vi "Get State.vi"(8 "error in (no error)":errorcluster, 11 "Tektronix Driver in":refnum<class "Tektronix Driver.lvclass">) -> (0 "error out":errorcluster, 1 "Data ready":bool, 2 "Armed":bool, 3 "Tektronix Driver out":refnum<class "Tektronix Driver.lvclass">, 4 "Availiable Samples":u32, 5 "Finished":bool)   [LabVIEW 2020, in "Tektronix Driver.lvclass"]
uses:
  Tektronix Driver.lvclass
  Tektronix Driver.lvclass/Tektronix Driver.ctl
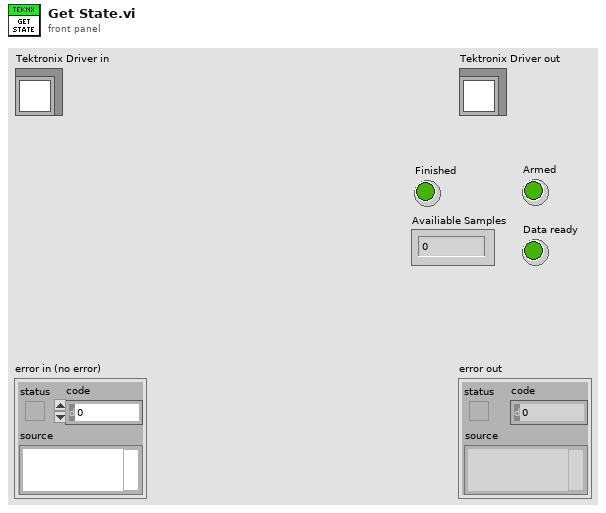
[diagram p1: front panel]
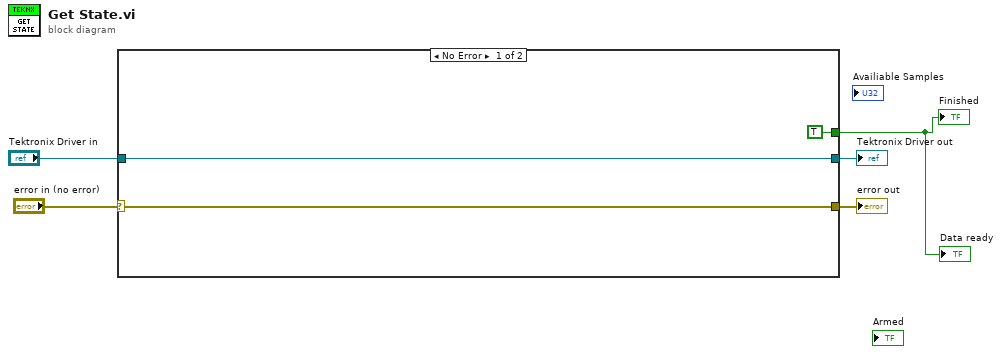
[diagram p0: block diagram]
diagram:
  n1 = case shown="No Error" "error in (no error)" {
    selector: "error in (no error)" -> [w8 w10]
    tunnel: [w8 w10] -> w4
    tunnel: [w7 w9] -> w2
    tunnel: "Tektronix Driver in" -> [w7 w9]
    tunnel: [TRUE _] -> w1
    frame No Error {
    }
    frame Error {
    }
  }
  "error out" <- w4
  "Tektronix Driver out" <- w2
  "Finished" <- w1
  "Data ready" <- w1
